vi "Stream Options.vi"(8 "error in (no error)":errorcluster, 11 "TCP Client in":refnum<class "TCP Client.lvclass">) -> (0 "error out":errorcluster, 3 "TCP Client out":refnum<class "TCP Client.lvclass">, 5 "Timeout ms":i32, 7 "TCP Mode":T1=enum."raw")   [LabVIEW 2020, in "Stream-TCP.lvlib" / "TCP Client.lvclass"]
uses:
  TCP Client.lvclass
  TCP Mode.ctl
  TCP Client.lvclass/TCP Client.ctl
  Stream-TCP.lvlib
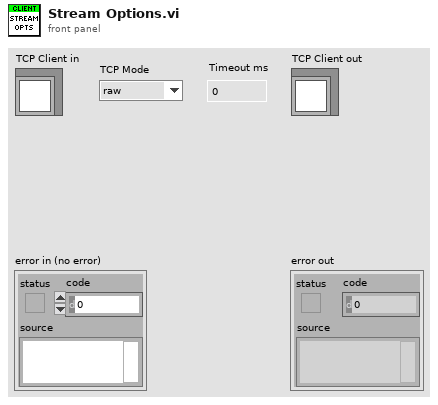
[diagram p1: front panel]
types:
  T1 = typedef "Stream-TCP.lvlib/TCP Mode.ctl" = enum16{"buffered", "raw"}
  T2 = typedef "Stream-TCP.lvlib/TCP Client.lvclass/Ref Data.ctl" = cluster{"TCP Connection":refnum<k5>, "TCP Stream":refnum<class "TCP Stream.lvclass">, "State":T3, "Connection Loop":refnum<vi>, "TCP Mode":T1, "Timeout ms":i32, "Server Connection":bool}
  T3 = typedef "Stream-TCP.lvlib/TCP Client.lvclass/Connection State.ctl" = enum16{"Closed", "Idle", "Connecting", "Connected", "Shutdown"}
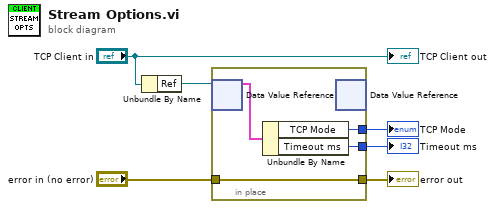
[diagram p0: block diagram]
diagram:
  n1 = Unbundle By Name("TCP Client in") -> ("Ref"=w6:refnum<data-value>)
  n2 = in-place {
    in-place-border: [w9] -> w3
    in-place-border: [w8] -> w4
    in-place-border: "error in (no error)" -> [w7]
    in-place-border: [w7] -> w1
    n3 = in-place-dvr #1(w6) -> (w10:T2)  [unwired: 1 out]
    n4 = Unbundle By Name(w10) -> ("TCP Mode"=w9:T1, "Timeout ms"=w8:i32)
    n5 = in-place-dvr #1() -> ()  [unwired: 1 in, 2 out]
  }
  "error out" <- w1
  "TCP Mode" <- w3
  "Timeout ms" <- w4
  "TCP Client out" <- "TCP Client in"
